vi "Update Front Panel.vi"(8 "error in (no error)":errorcluster, 11 "MediatorBusMonitor In":refnum<class "MediatorBusMonitor.lvclass">) -> (0 "error out":errorcluster, 3 "MediatorBusMonitor Out":refnum<class "MediatorBusMonitor.lvclass">)   [LabVIEW 2017, in "MyMediator.lvlib副本.lvlib" / "MediatorBusMonitor.lvclass"]
uses:
  MediatorBusMonitor/MediatorBusMonitor.lvclass
  MediatorBusMonitor/MediatorBusMonitor.lvclass/MediatorBusMonitor.ctl
  <vilib>/Composed/GPM Packages/lookup-table/Source/LookupTable/LookupTable.lvclass/LookupTable.ctl
  8fba652b-b38e-4eb6-874c-41f96ca6a9a0.vi
  <vilib>/Composed/GPM Packages/lookup-table/Source/LookupTable/Read Table Reference.vi
  <vilib>/Composed/GPM Packages/variant/Source/Scalar Data to String.vi
  <vilib>/Utility/Data Type/Get Type Information.vi
  <vilib>/Utility/Data Type/Get Refnum Information.vi
  <vilib>/Composed/GPM Packages/lookup-table/Source/LookupTable/LookupTable.lvclass
  <vilib>/Composed/GPM Packages/variant/Source/VariantExtensions.lvlib
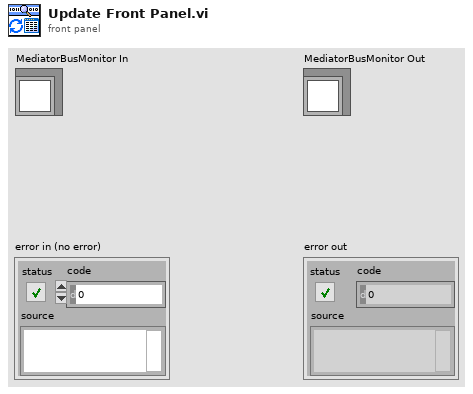
[diagram p1: front panel]
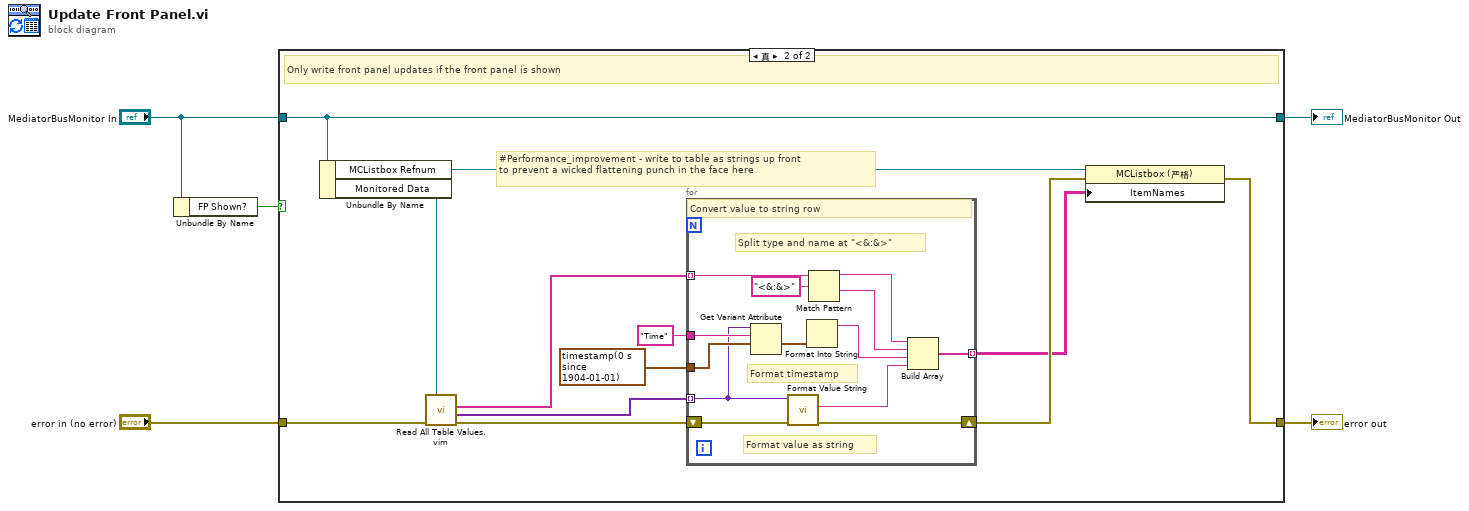
[diagram p0: block diagram]
diagram:
  n1 = Unbundle By Name("MediatorBusMonitor In") -> ("FP Shown?"=w3:bool)
  n2 = case shown="真" w3 {
    tunnel: "MediatorBusMonitor In" -> [w7 w12]
    tunnel: [w7 w12] -> w5
    tunnel: "error in (no error)" -> [w6 w16]
    tunnel: [w6 w13] -> w1
    frame False {
    }
    frame True {
      # "#Performance_improvement - write to table as strings up front\nto prevent a wicked flattening punch in the face here"
      # "Only write front panel updates if the front panel is shown"
      n3 = Unbundle By Name(w12) -> ("MCListbox Refnum"=w19:refnum<vi>, "Monitored Data"=w18:refnum<data-value>)
      n4 = call "Read All Table Values.vim"("error in (no error)"=w16, "LookupTable Reference"=w18) -> ("error out"=w15:errorcluster, "Values"=w17:variant[], "Names"=w11:string[])  [unwired: 6 in, 1 out]
      n5 = for {
        tunnel: w17 -> [w21] mode=indexing
        shift-right: [w22] -> w14
        shift-left: w15 -> [w23]
        tunnel: w11 -> [w29] mode=indexing
        tunnel: timestamp(0 s since 1904-01-01) -> [w31]
        tunnel: [w25] -> w9 mode=indexing
        tunnel: "Time" ("name") -> [w24]
        # "Format timestamp"
        # "Format value as string"
        # "Split type and name at \"<&:&>\""
        # "Convert value to string row"
        n6 = Get Variant Attribute(Variant=w21, name=w24, default value (empty Variant)=w31) -> (value=w30:timestamp)  [unwired: 1 in, 3 out]
        n7 = call <vilib>:"Format Value String.vi"("error in (no error)"=w23, "Data"=w21) -> ("error out"=w22:errorcluster, "Value as String"=w20:string)  [unwired: 8 in]
        n8 = Format Into String(w30) -> (resulting string=w32:string)  [unwired: 3 in, 1 out]
        n9 = Match Pattern(string=w29, regular expression="<&:&>" ("search string/char (-)")) -> (before substring=w27:string, after substring=w26:string)  [unwired: 1 in, 2 out]
        n10 = Build Array(w27, w26, w32, w20) -> (w25:string[])
      }
      n11 = property class="MCListbox (严格)"(reference=w19, error in=w14, "ItemNames"=w9) -> (error out=w13:errorcluster)  [unwired: 1 out]
    }
  }
  "MediatorBusMonitor Out" <- w5
  "error out" <- w1
